vi "niRFUtil RFHS Channelizer FineTuneResamplerRef CSG.vi"(0 "Resampler Ref":refnum<data-value>, 1 "Source Channelizer Ref":refnum<data-value>, 2 "Length":i32=-1, 3 "Channnel":i32, 4 "fs shift (ppm)":dbl, 5 "error in (no error)":errorcluster, 6 "Reset":bool, 7 "phase shift (samples)":dbl, 8 "Requested Output Samples":i32=-1, 10 "Benchmark Task":T1, 11 "CPU Context":string) -> (14 "Resampler Ref (out)":refnum<data-value>, 15 "Channel Data":csg[](array[numeric]), 19 "error out":errorcluster)   [LabVIEW 2015, in "niRFUtil.lvlib"]
uses:
  niRFUtil.lvlib
  Utilities/Benchmark/niRFUtil RFHS Benchmark Task.ctl
  Includes/niRFUtil RFHS Channelizer ChannelizerInfo CSG.ctl
  Includes/niRFUtil RFHS Channelizer FilterRef.ctl
  Includes/niRFUtil RFHS Channelizer ChannelizerBufferingMode.ctl
  Utilities/Data FIFO/niRFUtil RFHS FIFO Reference.ctl
  Utilities/Data FIFO/niRFUtil RFHS FIFO.ctl
  Includes/niRFUtil RFHS Channelizer ChannelizerType.ctl
  Includes/niRFUtil RFHS Channelizer ChannelizerFlags.ctl
  Includes/niRFUtil RFHS Channelizer ResamplerInfo CSG.ctl
  Includes/niRFUtil RFHS Channelizer ChannelizerErrors.ctl
  niRFUtil RFHS Channelizer AdjustDataSubsetSpecification.vi
  niRFUtil RFHS Channelizer ChannelizerHandleDllError.vi
  niRFUtil RFHS Channelizer ProcessCPUContext.vi
  Utilities/niRFUtil RFHS Util Dll Path.vi
  niRFUtil RFHS Channelizer FineTuneResamplerCheck CSG.vi
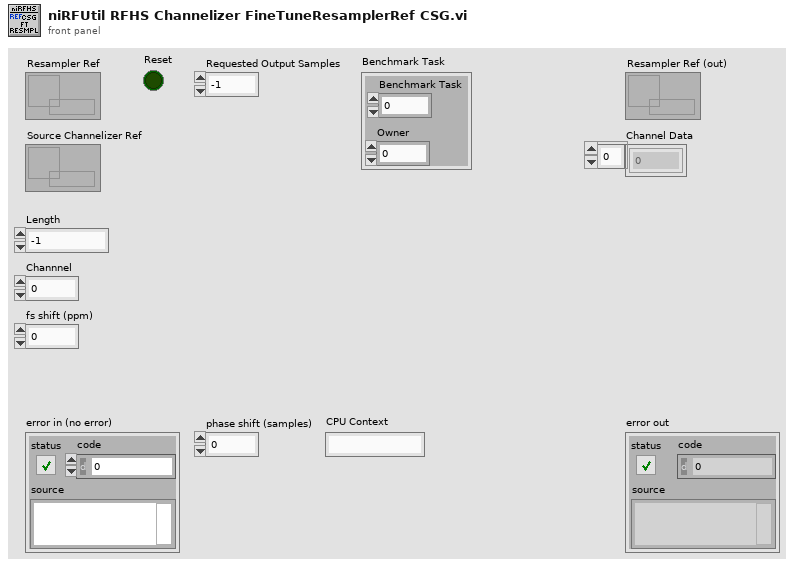
[diagram p1: front panel]
types:
  T1 = typedef "niRFUtil.lvlib/niRFUtil RFHS Benchmark Task.ctl" = cluster{"Benchmark Task":u64, "Owner":u32}
  T2 = typedef "niRFUtil.lvlib/niRFUtil RFHS Channelizer ChannelizerErrors.ctl" = enum32{"No Error", "Invalid Channel", "Internal Error", "Invalid Channel fs", "Invalid Phase Shift", "Invalid fs", "Invalid Number Of Channles", "Invalid FFT Channel fs", "Invalid Resampler Channel fs", "Not a 15kHz Multiple", "Invalid Channel fc", "Invalid passBW/stopBW", "Coerced Rejection", "Requires Internal Buffer", "Duplicated Destination Channel Name", "Configuration Format Error", "Illegal Execution state", "DLL not found", "DLL loading failure", "AVX instruction failure"}
  T3 = typedef "niRFUtil.lvlib/niRFUtil RFHS Channelizer ChannelizerInfo CSG.ctl" = cluster{"Filter LVRef":T4, "Mode":T5, "History":csg[], "Buffer":csg[], "FIFO":T6, "History Len":u32, "Float Cache":csg[], "Double Cache":cdb[], "Type":T8, "Resample Phase":dbl, "fft1Descriptors":u64[], "fft2Descriptors":u64[], "FFT tBuf":csg[], "guardBandLen":i32, "FFT History":csg[], "FFT History Len":u32, "FFTInitDone":u32, "FFT Filter LVRefs":T4[], "FFT fc Offs":u32[], "fft2Sizes":u32[], "BufferW":u32[], "BufferR":u32[], "Buff Off":u32[], "Phase0 (fshift)":dbl[], "Phase (fshift)":dbl[], "fs phase step":dbl[], "Resample Step":dbl, "Flags":T9, "Reset Cnt":i64, "Filter Pass":u32, "Stages":variant[]}
  T4 = typedef "niRFUtil.lvlib/niRFUtil RFHS Channelizer FilterRef.ctl" = cluster{"Ref":u64, "GUID":u64, "Upsample":i32, "Downsample":i32, "Size":i32, "Num Taps":i32}
  T5 = typedef "niRFUtil.lvlib/niRFUtil RFHS Channelizer ChannelizerBufferingMode.ctl" = enum32{"Unbuffered", "Finite", "Continuous"}
  T6 = typedef "niRFUtil.lvlib/niRFUtil RFHS FIFO Reference.ctl" = cluster{"Read Lock":refnum<data-value>, "Info":T7, "Write Lock":refnum<data-value>}
  T7 = typedef "niRFUtil.lvlib/niRFUtil RFHS FIFO.ctl" = cluster{"ID":u64, "Length":u32}
  T8 = typedef "niRFUtil.lvlib/niRFUtil RFHS Channelizer ChannelizerType.ctl" = enum32{"Auto", "Frequency Shift Only", "Resampler Only"}
  T9 = typedef "niRFUtil.lvlib/niRFUtil RFHS Channelizer ChannelizerFlags.ctl" = u32
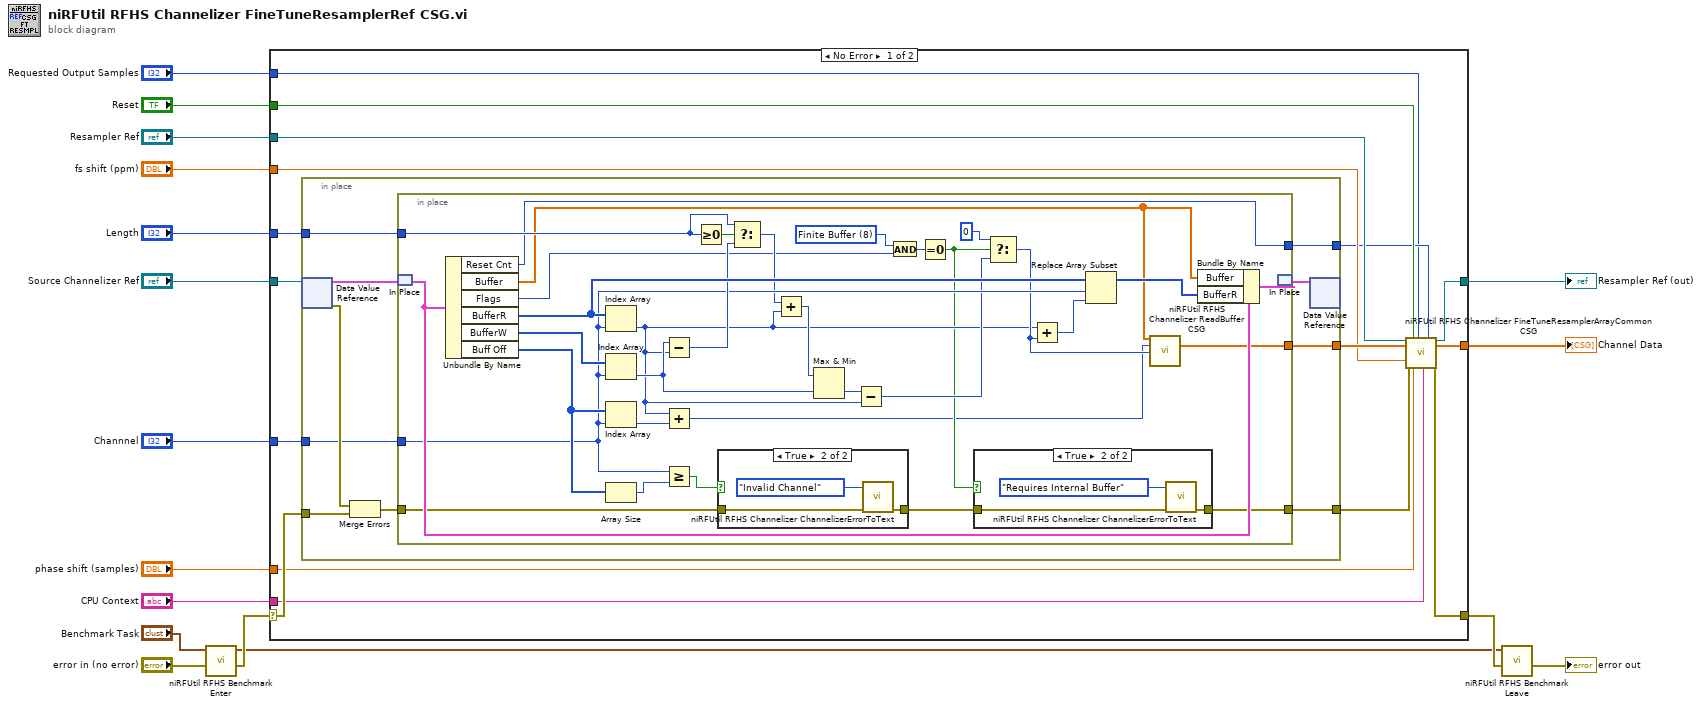
[diagram p0: block diagram]
diagram:
  n1 = call "niRFUtil RFHS Benchmark Enter.vi"("error in (no error)"="error in (no error)", "Benchmark Task (Parent)"="Benchmark Task") -> ("error out"=w14:errorcluster, "Benchmark Task (Self)"=w9:T1)  [unwired: 8 in]
  n2 = case shown="No Error" w14 {
    selector: w14 -> [w33 w86]
    tunnel: "Reset" -> [w25 _]
    tunnel: [w29 w86] -> w15
    tunnel: [w23 _] -> w11
    tunnel: "CPU Context" -> [w20 _]
    tunnel: "Source Channelizer Ref" -> [w32 _]
    tunnel: "Length" -> [w31 _]
    tunnel: "Channnel" -> [w30 _]
    tunnel: "Resampler Ref" -> [w28 w85]
    tunnel: "fs shift (ppm)" -> [w26 _]
    tunnel: "phase shift (samples)" -> [w21 _]
    tunnel: [w24 w85] -> w2
    tunnel: "Requested Output Samples" -> [w18 _]
    frame No Error {
      n3 = in-place {
        in-place-border: w33 -> [w39]
        in-place-border: w31 -> [w43]
        in-place-border: w30 -> [w38]
        in-place-border: [w37] -> w27
        in-place-border: [w36] -> w19
        in-place-border: [w34] -> w22
        n4 = in-place-dvr #1(w32) -> (w42:T3, w40:errorcluster)
        n5 = Merge Errors(w40, w39) -> (w35:errorcluster)
        n6 = in-place {
          in-place-border: w43 -> [w76]
          in-place-border: w38 -> [w60]
          in-place-border: [w61] -> w37
          in-place-border: [w44] -> w36
          in-place-border: w35 -> [w62]
          in-place-border: [w57] -> w34
          w49 = T9 8 items=["None"=0, "Skip Stage 1"=1, "FFT Stage"=2, "Frequency Shift"=4, "Finite Buffer"=8, "Reset"=16, "Input Len Estimate"=32, "C buffers"=64, "Input From Ref"=128] ("y")
          n7 = in-place-match #2(w42) -> (w74:T3)
          n8 = Unbundle By Name(w74) -> ("Reset Cnt"=w44:i64, "Buffer"=w45:csg[], "Flags"=w48:T9, "BufferR"=w71:u32[], "BufferW"=w75:u32[], "Buff Off"=w65:u32[])
          n9 = Index Array(array=w71, index=w60) -> (element=w51:u32)
          n10 = Index Array(array=w75, index=w60) -> (element=w67:u32)
          n11 = Index Array(array=w65, index=w60) -> (element=w66:u32)
          n12 = Array Size(array=w65) -> (size(s)=w64:i32)
          n13 = Subtract(x=w67, y=w51) -> (x-y=w68:u32)
          n14 = Add(x=w51, y=w66) -> (x+y=w46:u32)
          n15 = Greater Or Equal?(x=w60, y=w64) -> (x >= y?=w63:bool)
          n16 = Greater Or Equal To 0?(x=w76) -> (x >= 0?=w69:bool)
          n17 = case shown="True" w63 {
            tunnel: w62 -> [w81 w83]
            tunnel: [w81 w82] -> w58
            frame False {
            }
            frame True {
              n18 = call "niRFUtil RFHS Channelizer ChannelizerErrorToText.vi"("Error List"=niRFUtil_RFHS_Channelizer_ChannelizerErrors."Invalid Channel", "error in (no error)"=w83) -> ("error out"=w82:errorcluster)  [unwired: 13 in]
            }
          }
          n19 = Select(t=w76, s=w69, f=w68) -> (s? t:f=w50:u32)
          n20 = Add(x=w50, y=w51) -> (x+y=w70:u32)
          n21 = Max & Min(x=w70, y=w67) -> (min(x,y)=w56:u32)  [unwired: 1 out]
          n22 = Subtract(x=w56, y=w51) -> (x-y=w55:u32)
          n23 = And(x=w49, y=w48) -> (x .and. y?=w59:T9)
          n24 = Equal To 0?(x=w59) -> (x = 0?=w47:bool)
          n25 = case shown="True" w47 {
            tunnel: w58 -> [w77 w79]
            tunnel: [w77 w78] -> w57
            frame False {
            }
            frame True {
              n26 = call "niRFUtil RFHS Channelizer ChannelizerErrorToText.vi"("Error List"=niRFUtil_RFHS_Channelizer_ChannelizerErrors."Requires Internal Buffer", "error in (no error)"=w79) -> ("error out"=w78:errorcluster)  [unwired: 13 in]
            }
          }
          n27 = Select(t=u32 0, s=w47, f=w55) -> (s? t:f=w53:u32)
          n28 = Add(x=w51, y=w53) -> (x+y=w52:u32)
          n29 = Replace Array Subset(array=w71, new element=w52, index=w60) -> (w72:u32[])
          n30 = call "niRFUtil RFHS Channelizer ReadBuffer CSG.vi"("Buffer"=w45, "Index"=w46, "Length"=w53) -> ("Data"=w61:csg[])  [unwired: 12 in]
          n31 = Bundle By Name(cluster=w74, "Buffer"=w45, "BufferR"=w72) -> (w73:T3)
          n32 = in-place-match #2(w73) -> (w41:T3)
        }
        n33 = in-place-dvr #1(w41) -> ()  [unwired: 2 out]
      }
      n34 = call "niRFUtil RFHS Channelizer FineTuneResamplerArrayCommon CSG.vi"("Resampler Ref"=w28, "Data"=w27, "fs shift (ppm)"=w26, "error in (no error)"=w22, "Reset"=w25, "phase shift (samples)"=w21, "Requested Output Samples"=w18, "CPU Context"=w20, "Reset Cnt"=w19) -> ("Resampler Ref (out)"=w24:refnum<data-value>, "Resampled Data"=w23:csg[], "error out"=w29:errorcluster)  [unwired: 6 in, 2 out]
    }
    frame Error {
    }
  }
  "Channel Data" <- w11
  "Resampler Ref (out)" <- w2
  n35 = call "niRFUtil RFHS Benchmark Leave.vi"("error in (no error)"=w15, "Benchmark Task Self"=w9) -> ("error out"=→"error out":errorcluster)  [unwired: 8 in, 1 out]
